vi "Get Exclusive Access.vi"(0 "semaphore":T1, 1 "ms timeout (30000)":i32=30000, 2 "error in (no error)":errorcluster) -> (7 "error out":errorcluster)   [LabVIEW 2018, in "3458A Virtual Digitizer.lvlib" / "3458A Digitizing Low Levels.lvlib"]
doc: "Gains exclusive access usign semaphore. It is used to ensure only one instance of this driver accesses the bus at thse same time. \nIf the named semaphore is not found, it ignores the error. The sempahore must be created first! Once the exclusive access is not needed, release it!"
uses:
  3458A Digitizing Low Levels.lvlib
  <vilib>/Utility/error.llb/Error Cluster From Error Code.vi
  <vilib>/ErrorRing/Error Ring.xnode
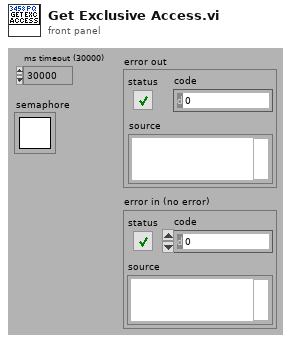
[diagram p1: front panel]
types:
  T1 = typedef "Semaphore RefNum" = refnum<k1>
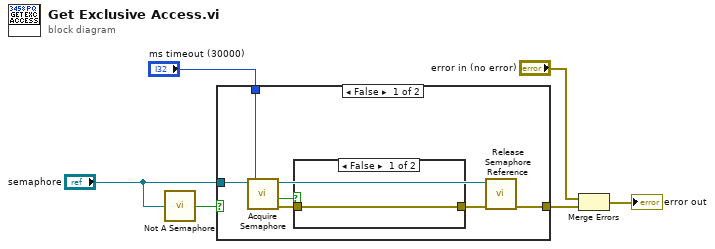
[diagram p0: block diagram]
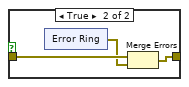
[diagram p2: hidden frame]
diagram:
  n1 = call <vilib>:"Not A Semaphore.vi"("semaphore"="semaphore") -> ("not a semaphore"=w1:bool)
  n2 = case shown="False" w1 {
    tunnel: "semaphore" -> [w13 _]
    tunnel: "ms timeout (30000)" -> [w12 _]
    tunnel: [w8 _] -> w5
    frame False {
      n3 = call <vilib>:"Acquire Semaphore.vi"("ms timeout (-1)"=w12, "semaphore"=w13) -> ("error out"=w11:errorcluster, "timed out"=w10:bool, "semaphore out"=w7:T1)  [unwired: 3 in]
      n4 = case shown="False" w10 {
        tunnel: w11 -> [w14 w17]
        tunnel: [w14 w15] -> w9
        frame False {
        }
        frame True {
          n5 = xnode "Error Ring"() -> ("error out"=w16:errorcluster)
          n6 = Merge Errors(w17, w16) -> (w15:errorcluster)
        }
      }
      n7 = call <vilib>:"Release Semaphore Reference.vi"("error in (no error)"=w9, "semaphore"=w7) -> ("error out"=w8:errorcluster)  [unwired: 8 in, 1 out]
    }
    frame True {
    }
  }
  n8 = Merge Errors("error in (no error)", w5) -> (→"error out":errorcluster)
